vi "Project2FrontPanel_withActionEngine.vi"() -> ()   [LabVIEW 2018]
uses:
  StateVariable.ctl
  DIO_Action(enum).ctl
panel:
  out "Code Entry Buttons":bool[](array[boolean])
  out "Reset":bool
  out "State":T1
  out "Clock":bool
  in  "STOP":bool
  out "Lock \nStatus":bool[](array[boolean])
  # "B0"
  # "Locked"
  # "C"
  # "B"
  # "B1"
  # "A"
  # "B2"
  # "B3"
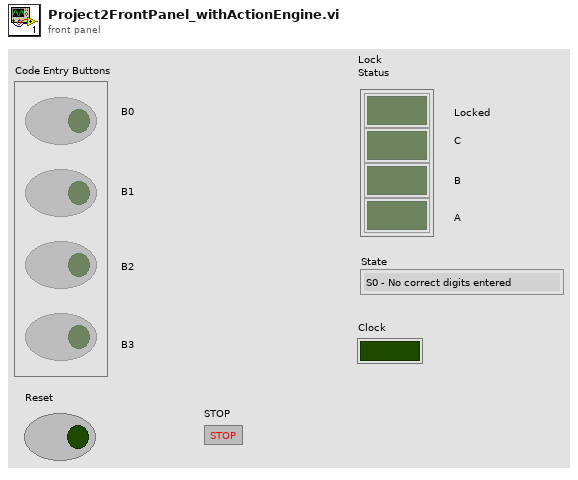
[diagram p1: front panel]
types:
  T1 = typedef "StateVariable.ctl" = enum16{"S0 - No correct digits entered", "S1 - One correct digit entered", "S2 - Two correct digits entered", "S3 - Three correct digits entered.", "S4 - Code entered"}
  T2 = typedef "DIO_Action(enum).ctl" = enum16{"Initialize", "Read Code Entry Buttons", "Read Reset Button", "Write Lock Status", "Write Clock", "Release"}
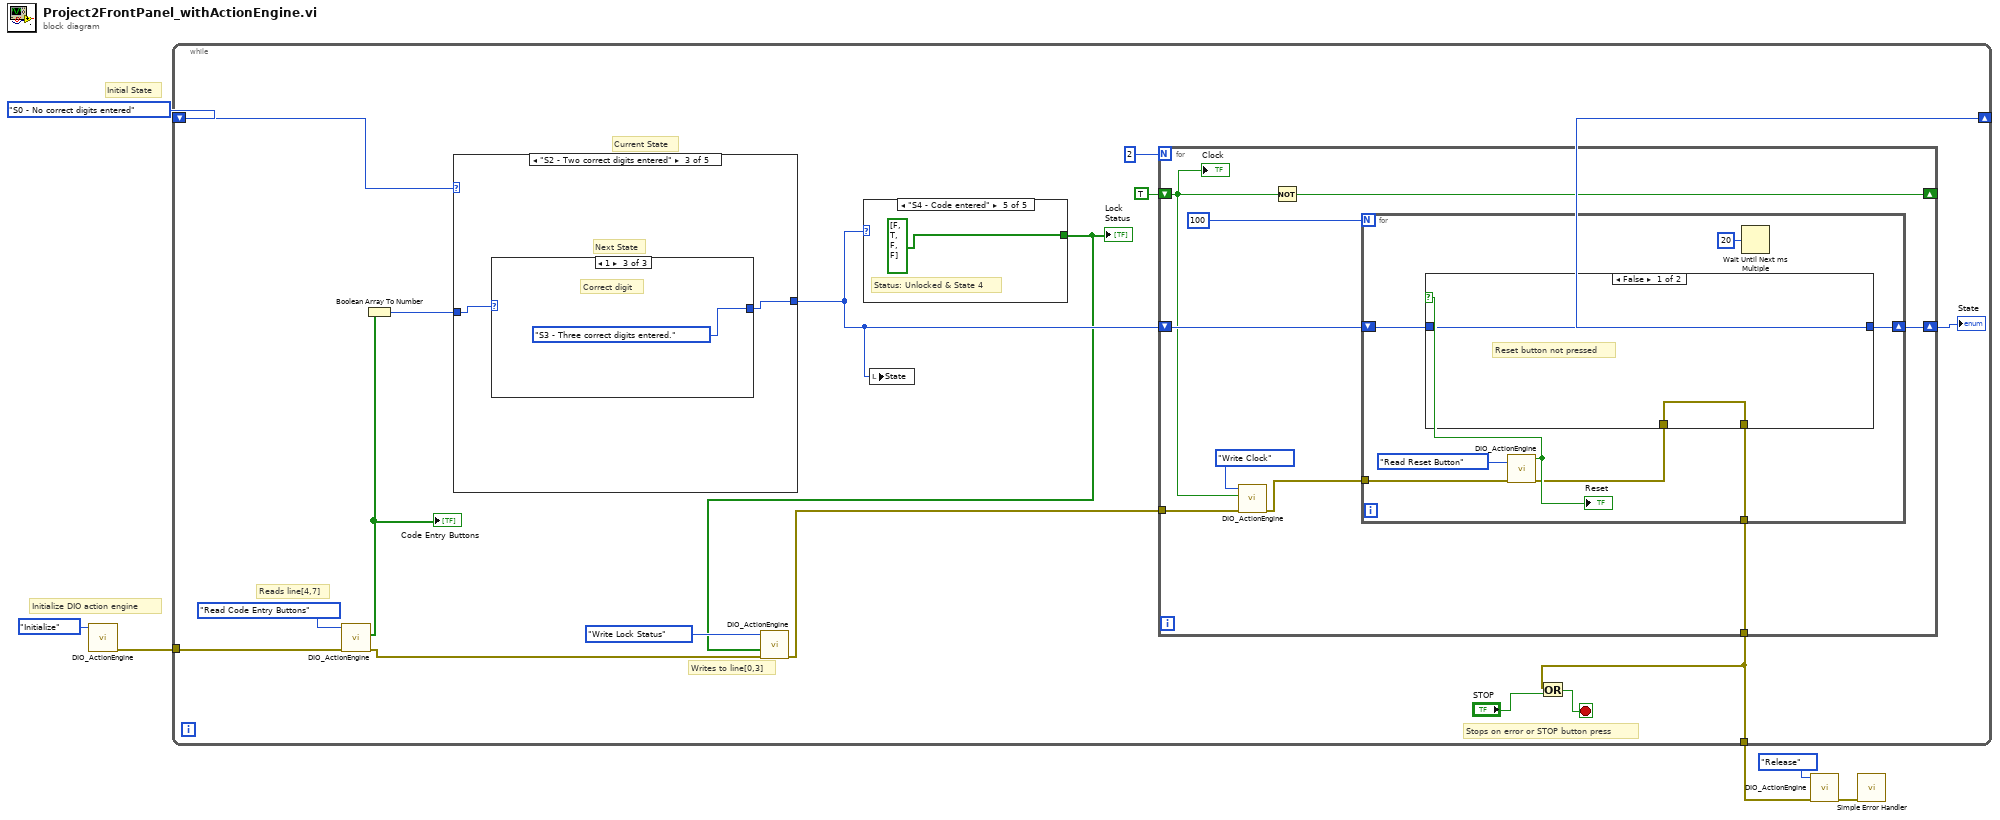
[diagram p0: block diagram]
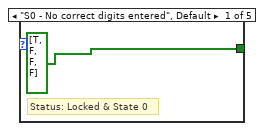
[diagram p2: hidden frame]
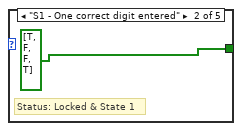
[diagram p3: hidden frame]
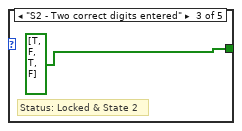
[diagram p4: hidden frame]
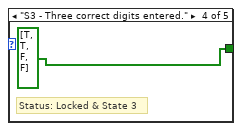
[diagram p5: hidden frame]
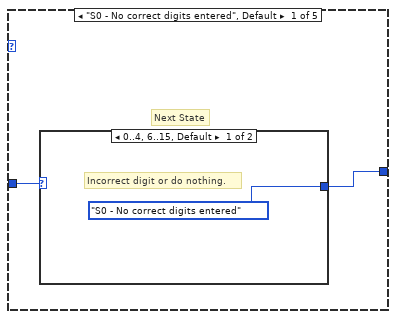
[diagram p6: hidden frame]
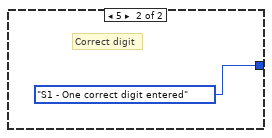
[diagram p7: hidden frame]
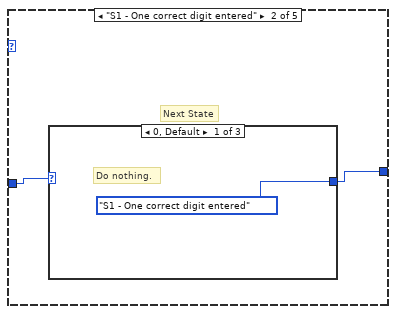
[diagram p8: hidden frame]
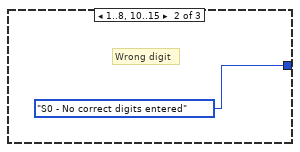
[diagram p9: hidden frame]
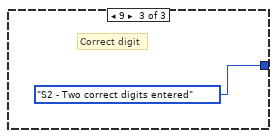
[diagram p10: hidden frame]
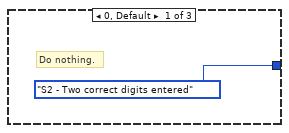
[diagram p11: hidden frame]
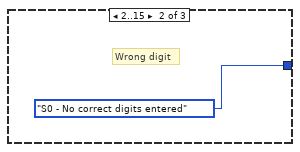
[diagram p12: hidden frame]
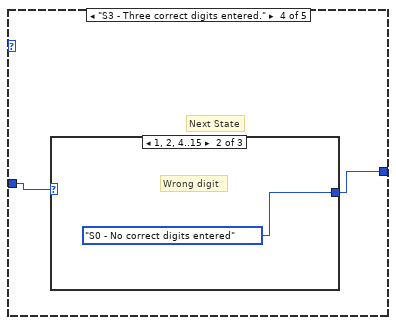
[diagram p13: hidden frame]
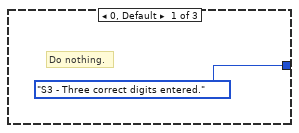
[diagram p14: hidden frame]
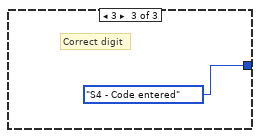
[diagram p15: hidden frame]
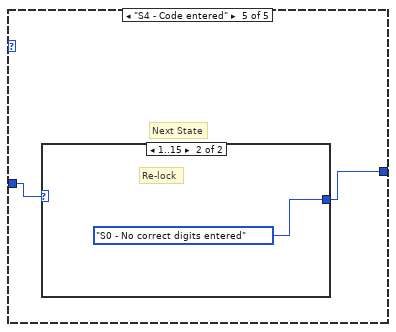
[diagram p16: hidden frame]
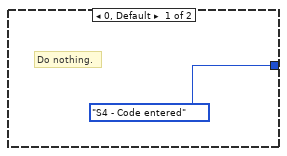
[diagram p17: hidden frame]
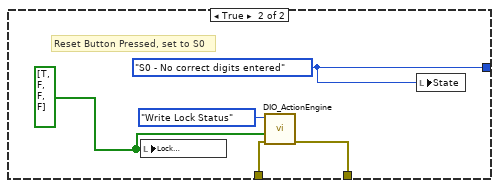
[diagram p18: hidden frame]
diagram:
  # "Initialize DIO action engine"
  # "Initial State"
  n1 = call "DIO_ActionEngine.vi"("DIO Action"=DIO_Action(enum)."Initialize") -> ("error out"=w4:errorcluster)  [unwired: 8 in, 2 out]
  n2 = while {
    shift-right: [w20] -> _
    shift-left: StateVariable."S0 - No correct digits entered" ("State") -> [w19]
    tunnel: w4 -> [w17]
    tunnel: [w8] -> w3
    stop <- w9 stop-if-true
    # "Stops on error or STOP button press"
    # "Writes to line[0,3]"
    # "Current State"
    # "Reads line[4,7]"
    n3 = call "DIO_ActionEngine.vi"("error in"=w17, "DIO Action"=DIO_Action(enum)."Read Code Entry Buttons") -> ("error out"=w13:errorcluster, "System Inputs"=w15:bool[])  [unwired: 7 in, 1 out]
    "Code Entry Buttons" <- w15
    n4 = Boolean Array To Number(Boolean array=w15) -> (number=w18:u32)
    n5 = case shown="\"S2 - Two correct digits entered\"" w19 {
      tunnel: [w29 w32 w37 w42 w48] -> w14
      tunnel: w18 -> [w28 w33 w38 w43 w47]
      frame "S0 - No correct digits entered", Default {
        # "Next State"
        n6 = case shown="0..4, 6..15, Default" w28 {
          tunnel: [StateVariable."S0 - No correct digits entered" ("State") StateVariable."S1 - One correct digit entered" ("State")] -> w29
          frame 0..4, 6..15, Default {
            # "Incorrect digit or do nothing."
          }
          frame 5 {
            # "Correct digit"
          }
        }
      }
      frame "S1 - One correct digit entered" {
        # "Next State"
        n7 = case shown="0, Default" w33 {
          tunnel: [StateVariable."S1 - One correct digit entered" ("State") StateVariable."S0 - No correct digits entered" ("State") StateVariable."S2 - Two correct digits entered" ("State")] -> w32
          frame 0, Default {
            # "Do nothing."
          }
          frame 1..8, 10..15 {
            # "Wrong digit"
          }
          frame 9 {
            # "Correct digit"
          }
        }
      }
      frame "S2 - Two correct digits entered" {
        # "Next State"
        n8 = case shown="1" w38 {
          tunnel: [StateVariable."S2 - Two correct digits entered" ("State") StateVariable."S0 - No correct digits entered" ("State") StateVariable."S3 - Three correct digits entered." ("State")] -> w37
          frame 0, Default {
            # "Do nothing."
          }
          frame 2..15 {
            # "Wrong digit"
          }
          frame 1 {
            # "Correct digit"
          }
        }
      }
      frame "S3 - Three correct digits entered." {
        # "Next State"
        n9 = case shown="1, 2, 4..15" w43 {
          tunnel: [StateVariable."S3 - Three correct digits entered." ("State") StateVariable."S0 - No correct digits entered" ("State") StateVariable."S4 - Code entered" ("State")] -> w42
          frame 0, Default {
            # "Do nothing."
          }
          frame 1, 2, 4..15 {
            # "Wrong digit"
          }
          frame 3 {
            # "Correct digit"
          }
        }
      }
      frame "S4 - Code entered" {
        # "Next State"
        n10 = case shown="1..15" w47 {
          tunnel: [StateVariable."S4 - Code entered" ("State") StateVariable."S0 - No correct digits entered" ("State")] -> w48
          frame 0, Default {
            # "Do nothing."
          }
          frame 1..15 {
            # "Re-lock"
          }
        }
      }
    }
    n11 = case shown="\"S4 - Code entered\"" w14 {
      tunnel: [bool[] [TRUE, FALSE, FALSE, FALSE] bool[] [TRUE, FALSE, FALSE, TRUE] bool[] [TRUE, FALSE, TRUE, FALSE] bool[] [TRUE, TRUE, FALSE, FALSE] bool[] [FALSE, TRUE, FALSE, FALSE]] -> w7
      frame "S0 - No correct digits entered", Default {
        # "Status: Locked & State 0"
      }
      frame "S1 - One correct digit entered" {
        # "Status: Locked & State 1"
      }
      frame "S2 - Two correct digits entered" {
        # "Status: Locked & State 2"
      }
      frame "S3 - Three correct digits entered." {
        # "Status: Locked & State 3"
      }
      frame "S4 - Code entered" {
        # "Status: Unlocked & State 4"
      }
    }
    "Lock \nStatus" <- w7
    n12 = call "DIO_ActionEngine.vi"("error in"=w13, "System Outputs"=w7, "DIO Action"=DIO_Action(enum)."Write Lock Status") -> ("error out"=w11:errorcluster)  [unwired: 6 in, 2 out]
    n13 = local write "State"(w14) -> ()
    n14 = for {
      N: 2 -> [_]
      shift-right: [w58] -> _
      shift-left: TRUE -> [w53]
      shift-right: [w56] -> w20
      shift-left: w14 -> [w57]
      tunnel: w11 -> [w55]
      tunnel: [w51] -> w8
      n15 = call "DIO_ActionEngine.vi"("error in"=w55, "Clock"=w53, "DIO Action"=DIO_Action(enum)."Write Clock") -> ("error out"=w52:errorcluster)  [unwired: 6 in, 2 out]
      n16 = Not(x=w53) -> (.not. x?=w58:bool)
      n17 = for {
        N: 100 -> [_]
        shift-right: [w65] -> w56
        shift-left: w57 -> [w66]
        tunnel: w52 -> [w64]
        tunnel: [w60] -> w51
        n18 = call "DIO_ActionEngine.vi"("error in"=w64, "DIO Action"=DIO_Action(enum)."Read Reset Button") -> ("error out"=w61:errorcluster, "Reset"=w62:bool)  [unwired: 7 in, 1 out]
        "Reset" <- w62
        n19 = case shown="False" w62 {
          tunnel: w66 -> [w69 _]
          tunnel: [w69 w74] -> w65
          tunnel: w61 -> [w68 w73]
          tunnel: [w68 w72] -> w60
          frame False {
            # "Reset button not pressed"
          }
          frame True {
            w70 = bool[] [TRUE, FALSE, FALSE, FALSE]
            w74 = StateVariable."S0 - No correct digits entered" ("State")
            # "Reset Button Pressed, set to S0"
            n20 = local write "Lock \nStatus"(w70) -> ()
            n21 = call "DIO_ActionEngine.vi"("error in"=w73, "System Outputs"=w70, "DIO Action"=DIO_Action(enum)."Write Lock Status") -> ("error out"=w72:errorcluster)  [unwired: 6 in, 2 out]
            n22 = local write "State"(w74) -> ()
          }
        }
        n23 = Wait Until Next ms Multiple(millisecond multiple=u32 20) -> ()  [unwired: 1 out]
      }
      "Clock" <- w53
    }
    "State" <- w20
    n24 = Or(x=w8, y="STOP") -> (x .or. y?=w9:bool)
  }
  n25 = call "DIO_ActionEngine.vi"("error in"=w3, "DIO Action"=DIO_Action(enum)."Release") -> ("error out"=w1:errorcluster)  [unwired: 7 in, 2 out]
  n26 = call <vilib>:"Simple Error Handler.vi"("error in (no error)"=w1) -> ()  [unwired: 4 in, 5 out]
